vi "Check for Input Register Mapping Conflicts.vi"(8 "error in (no error)":errorcluster, 11 "Group Ref in":T1 format="%.0x") -> (0 "error out":errorcluster, 1 "Conflicts?":bool, 2 "Conflicts":T2(array[cluster]), 3 "Coil Group Ref out":T1 format="%.0x")   [LabVIEW 2019, in "Modbus Master System Explorer.lvlib"]
uses:
  Modbus Master System Explorer.lvlib
  <vilib>/NI VeriStand/Custom Device API/Custom Device Item Ref.ctl
  Modbus Type.ctl
  Shared/Modbus Master Shared.lvlib
  <vilib>/NI VeriStand/Custom Device API/Custom Device API.lvlib
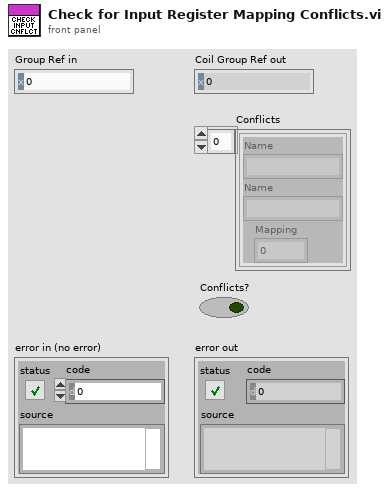
[diagram p1: front panel]
types:
  T1 = typedef "Custom Device API.lvlib/Custom Device Item Ref.ctl" = u64
  T2 = cluster{"Name":string, "Name":string, "Mapping":u16}[]
  T3 = typedef "Modbus Master Shared.lvlib/Modbus Type.ctl" = enum16{"Coil", "Discrete Input", "Holding Register", "Input Register"}
  T4 = typedef "Modbus Master Shared.lvlib/Mapping.ctl" = cluster{"DataType":T5, "Starting Address":u16, "Sub-Index (Bool)":u16, "VS Reference":T1}
  T5 = typedef "Modbus Master Shared.lvlib/DataType.ctl" = enum16{"Double", "Single", "I64", "I32", "I16", "I8", "U64", "U32", "U16", "U8", "Boolean"}
  T6 = typedef "Custom Device API.lvlib/Custom Device Item Info.ctl" = cluster{"Name":string, "Is Channel":bool, "GUID":string, "Is Waveform":bool}
  T7 = cluster{"Name":string, "Name":string, "Mapping":u16}
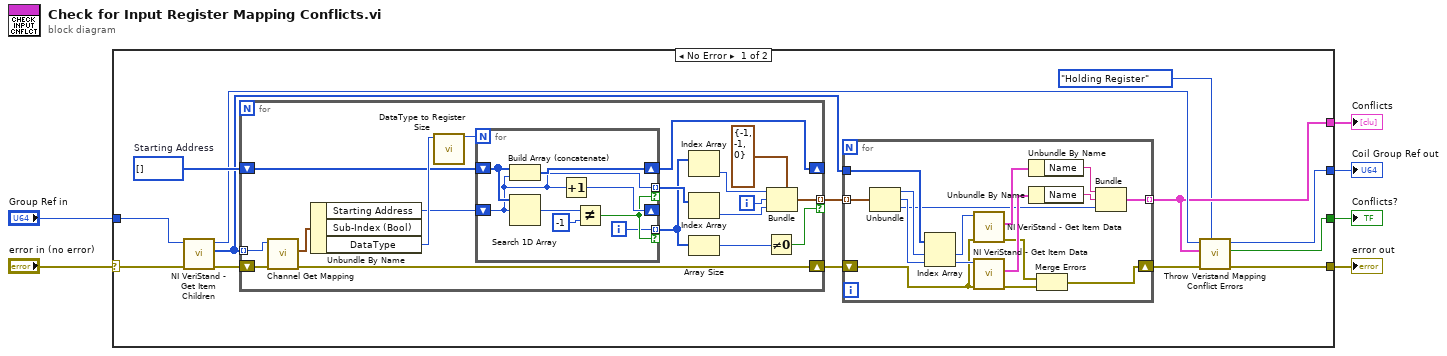
[diagram p0: block diagram]
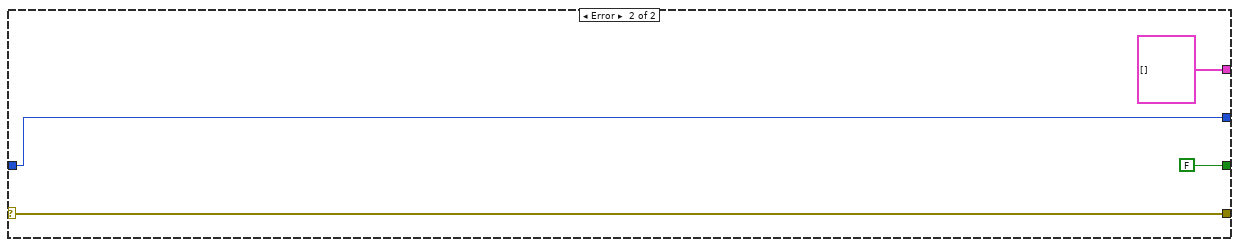
[diagram p2: hidden frame]
diagram:
  n1 = case shown="No Error" "error in (no error)" {
    selector: "error in (no error)" -> [w18 w64]
    tunnel: "Group Ref in" -> [w19 w66]
    tunnel: [w17 w66] -> w4
    tunnel: [w15 T2 []] -> w3
    tunnel: [w13 w64] -> w2
    tunnel: [w12 FALSE ("Conflicts?")] -> w1
    frame No Error {
      w20 = u16[] []  # Starting Address
      n2 = call <vilib>:"NI VeriStand - Get Item Children.vi"("error in (no error)"=w18, "Item Ref in"=w19) -> ("error out"=w9:errorcluster, "Child Refs"=w10:T1[], "Item Ref out"=w16:T1)  [unwired: 6 in, 1 out]
      n3 = for {
        shift-right: [w47] -> _
        shift-left: w20 -> [w48]
        tunnel: [w53] -> w8 mode=indexing if=w45
        tunnel: w10 -> [w39] mode=indexing
        shift-right: [w37] -> w7
        shift-left: w9 -> [w38]
        i -> [w52]
        n4 = call "Channel Get Mapping.vi"("error in (no error)"=w38, "Item Ref in"=w39) -> ("error out"=w37:errorcluster, "Mapping"=w40:T4)  [unwired: 7 in, 1 out]
        n5 = Unbundle By Name(w40) -> ("Starting Address"=w49:u16, "DataType"=w51:T5)  [unwired: 1 out]
        n6 = call "DataType to Register Size.vi"("DataType"=w51) -> ("Registers"=w50:i32)  [unwired: 9 in, 1 out]
        n7 = for {
          N: w50 -> [_]
          shift-right: [w60] -> w47
          shift-left: w48 -> [w62]
          shift-right: [w61] -> _
          shift-left: w49 -> [w57]
          tunnel: [w55] -> w42 mode=indexing if=w56
          tunnel: [w57] -> w44 mode=indexing if=w56
          i -> [w55]
          n8 = Build Array (concatenate)(w62, w57) -> (w60:u16[])
          n9 = Search 1D Array(1D array=w62, element=w57) -> (index of element=w58:i32)  [unwired: 1 in]
          n10 = Increment(x=w57) -> (x+1=w61:u16)
          n11 = Not Equal?(x=w58, y=-1) -> (x != y?=w56:bool)
        }
        n12 = Index Array(array=w42) -> (element=w41:i32)  [unwired: 1 in]
        n13 = Index Array(array=w44) -> (element=w43:u16)  [unwired: 1 in]
        n14 = Array Size(array=w42) -> (size(s)=w46:i32)
        n15 = Not Equal To 0?(x=w46) -> (x != 0?=w45:bool)
        n16 = Bundle(cluster=cluster{"y":i32, "y 2":i32, "Mapping":u16} {"y"=-1, "y 2"=-1, "Mapping"=0} ("Conflicting Indices"), "y"=w41, "y 2"=w52, "Mapping"=w43) -> (w53:cluster{"y":i32, "y 2":i32, "Mapping":u16})
      }
      n17 = for {
        tunnel: w8 -> [w36] mode=indexing
        tunnel: w10 -> [w35]
        tunnel: [w26] -> w15 mode=indexing
        shift-right: [w21] -> w14
        shift-left: w7 -> [w24]
        n18 = Unbundle(w36) -> ("y"=w34:i32, "y 2"=w33:i32, "Mapping"=w25:u16)
        n19 = Index Array(array=w35, index #1=w34, index #2=w33) -> (element #1=w32:T1, element #2=w31:T1)
        n20 = call <vilib>:"NI VeriStand - Get Item Data.vi"("error in (no error)"=w24, "Item Ref in"=w32) -> ("error out"=w23:errorcluster, "Item Info"=w30:T6)  [unwired: 8 out]
        n21 = call <vilib>:"NI VeriStand - Get Item Data.vi"("error in (no error)"=w24, "Item Ref in"=w31) -> ("error out"=w22:errorcluster, "Item Info"=w29:T6)  [unwired: 8 out]
        n22 = Unbundle By Name(w30) -> ("Name"=w28:string)
        n23 = Unbundle By Name(w29) -> ("Name"=w27:string)
        n24 = Merge Errors(w23, w22) -> (w21:errorcluster)
        n25 = Bundle("Name"=w28, "Name"=w27, "Mapping"=w25) -> (w26:T7)  [unwired: 1 in]
      }
      n26 = call "Throw Veristand Mapping Conflict Errors.vi"("Type"=Modbus_Type."Holding Register", "error in (no error)"=w14, "Conflicts In"=w15, "Item Ref in"=w16) -> ("error out"=w13:errorcluster, "Conflicts?"=w12:bool, "Node Ref out"=w17:T1)  [unwired: 5 in]
    }
    frame Error {
    }
  }
  "Conflicts?" <- w1
  "Conflicts" <- w3
  "Coil Group Ref out" <- w4
  "error out" <- w2
